vi "Init GU Selection.vi"(7 "Curr Cal Cfg In":T1, 8 "error in":errorcluster, 10 "Latest Cal Cfg":T1, 11 "Config Data":T2(array[cluster])) -> (0 "error out":errorcluster, 2 "Curr Cal Cfg Out":T1, 3 "Config Data Out":T2(array[cluster]))   [LabVIEW 2020, in "GUCalibration2.lvlib"]
uses:
  GUCalibration2.lvlib
  Controls/Config Data Type.ctl
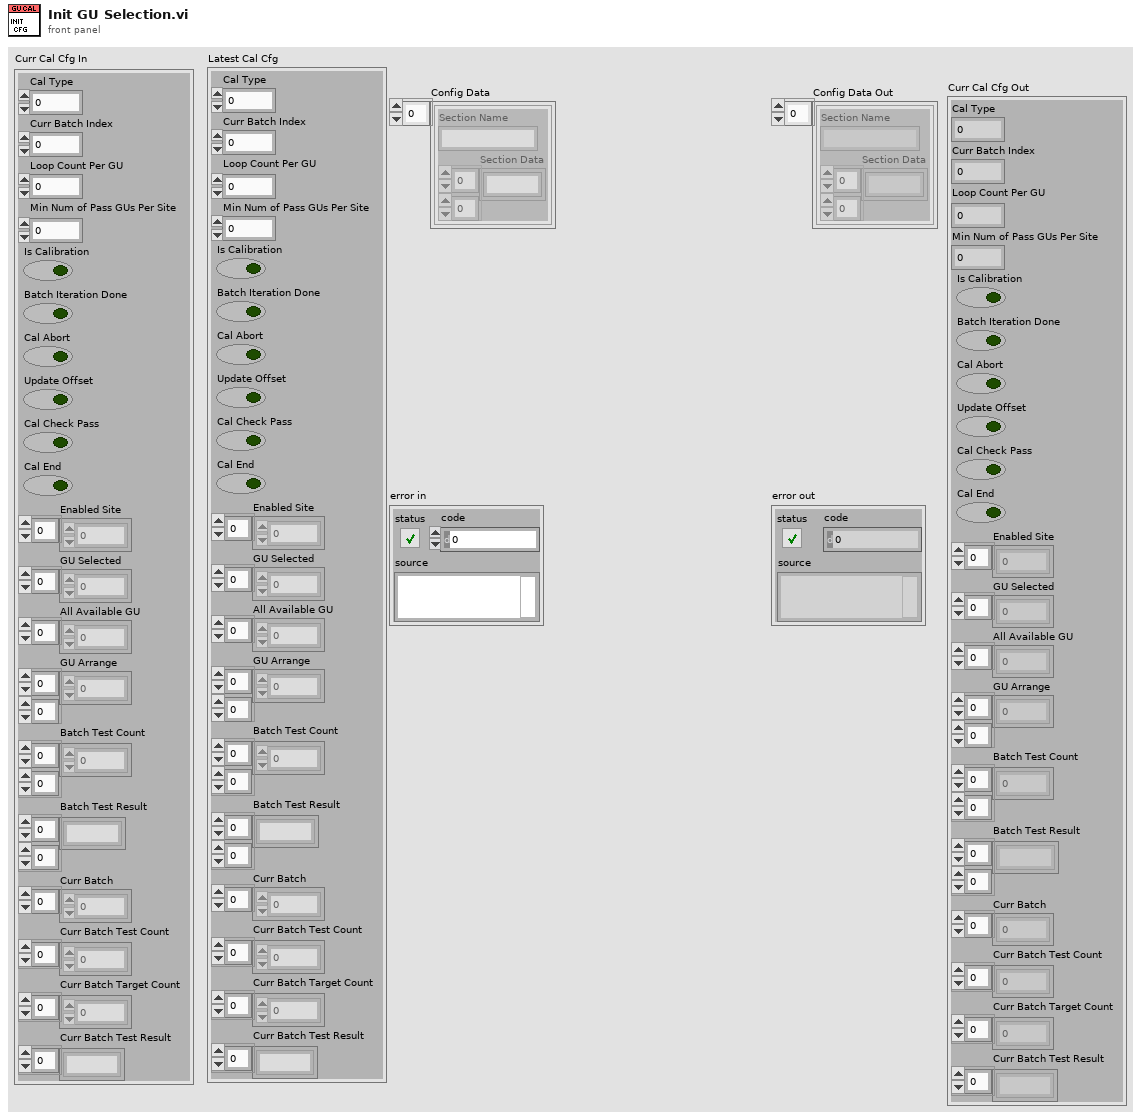
[diagram p1: front panel]
types:
  T1 = typedef "GUCalibration2.lvlib/Config Data Type.ctl" = cluster{"Cal Type":i32, "Curr Batch Index":i32, "Loop Count Per GU":i32, "Min Num of Pass GUs Per Site":i32, "Is Calibration":bool, "Batch Iteration Done":bool, "Cal Abort":bool, "Update Offset":bool, "Cal Check Pass":bool, "Cal End":bool, "Enabled Site":i32[], "GU Selected":i32[], "All Available GU":i32[], "GU Arrange":i32[][], "Batch Test Count":i32[][], "Batch Test Result":string[][], "Curr Batch":i32[], "Curr Batch Test Count":i32[], "Curr Batch Target Count":i32[], "Curr Batch Test Result":string[]}
  T2 = cluster{"Section Name":string, "Section Data":string[][]}[]
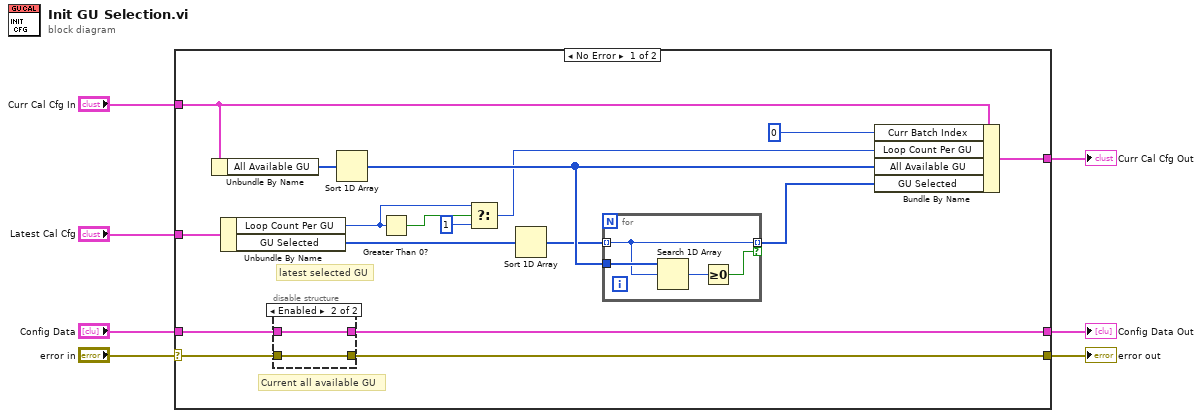
[diagram p0: block diagram]
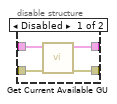
[diagram p2: hidden frame]
diagram:
  n1 = case shown="No Error" "error in" {
    selector: "error in" -> [w21 w36]
    tunnel: [w19 w36] -> w7
    tunnel: [w24 _] -> w5
    tunnel: "Latest Cal Cfg" -> [w12 _]
    tunnel: "Config Data" -> [w22 w35]
    tunnel: [w18 w35] -> w2
    tunnel: "Curr Cal Cfg In" -> [w14 _]
    frame No Error {
      # "latest selected GU"
      # "Current all available GU"
      n2 = Unbundle By Name(w14) -> ("All Available GU"=w13:i32[])
      n3 = Unbundle By Name(w12) -> ("Loop Count Per GU"=w10:i32, "GU Selected"=w16:i32[])
      n4 = disable-structure shown="Enabled" {
        disable-tunnel: w22 -> [w28 w30]
        disable-tunnel: w21 -> [w27 w29]
        disable-tunnel: [w26 w29] -> w19
        disable-tunnel: [w25 w30] -> w18
        frame Disabled {
          n5 = call "Get Current Available GU.vi"("error in"=w27, "Config Data"=w28) -> ("error out"=w26:errorcluster, "Config Data dup"=w25:T2)  [unwired: 7 in, 1 out]
        }
        frame Enabled {
        }
      }
      n6 = Sort 1D Array(array=w13) -> (sorted array=w17:i32[])
      n7 = Greater Than 0?(x=w10) -> (x > 0?=w11:bool)
      n8 = Select(t=w10, s=w11, f=1 ("Curr GU Index")) -> (s? t:f=w8:i32)
      n9 = Sort 1D Array(array=w16) -> (sorted array=w15:i32[])
      n10 = for {
        tunnel: w15 -> [w32] mode=indexing
        tunnel: w17 -> [w34]
        tunnel: [w32] -> w20 mode=indexing if=w31
        n11 = Search 1D Array(1D array=w34, element=w32) -> (index of element=w33:i32)  [unwired: 1 in]
        n12 = Greater Or Equal To 0?(x=w33) -> (x >= 0?=w31:bool)
      }
      n13 = Bundle By Name(cluster=w14, "Curr Batch Index"=0 ("Curr GU Index"), "Loop Count Per GU"=w8, "All Available GU"=w17, "GU Selected"=w20) -> (w24:T1)
    }
    frame Error {
    }
  }
  "error out" <- w7
  "Curr Cal Cfg Out" <- w5
  "Config Data Out" <- w2
